vi "Map(For).vi"(8 "error in (no error)":errorcluster, 10 "Step":dbl, 11 "Map":refnum<vi>[](array[refnum])) -> (0 "error out":errorcluster)   [LabVIEW 2010]
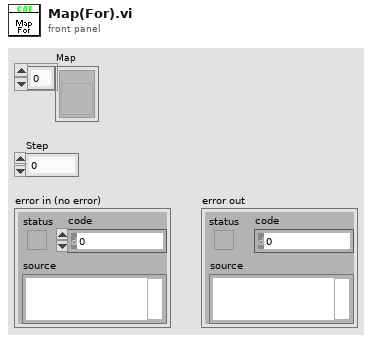
[diagram p1: front panel]
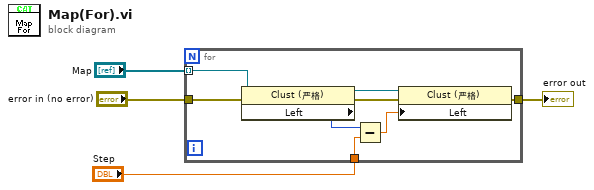
[diagram p0: block diagram]
diagram:
  n1 = for {
    tunnel: "Map" -> [w12] mode=indexing
    tunnel: [w9] -> w3
    tunnel: "error in (no error)" -> [w6]
    tunnel: "Step" -> [w5]
    n2 = property class="Clust (严格)"(reference=w12, error in=w6) -> (reference out=w11:refnum<vi>, error out=w10:errorcluster, "Left"=w7:i32)
    n3 = Subtract(x=w7, y=w5) -> (x-y=w8:dbl)
    n4 = property class="Clust (严格)"(reference=w11, error in=w10, "Left"=w8) -> (error out=w9:errorcluster)  [unwired: 1 out]
  }
  "error out" <- w3
